vi "Date_to_Seconds.vi"() -> ()   [LabVIEW 2020]
panel:
  out "Resultat en second":dbl
  in  "Secondes":dbl
  in  "Minutes":dbl
  in  "Heures":dbl
  in  "Jours":dbl
  in  "Mois":dbl
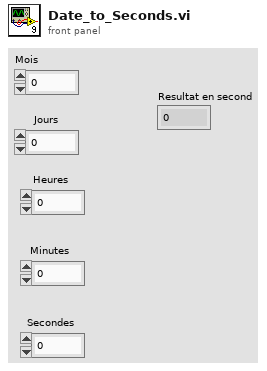
[diagram p1: front panel]
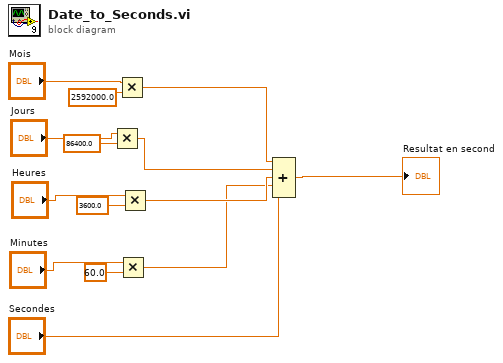
[diagram p0: block diagram]
diagram:
  n1 = Multiply(x="Jours", y=86400.0) -> (x*y=w5:dbl)
  n2 = Multiply(x="Mois", y=2592000.0) -> (x*y=w6:dbl)
  n3 = Multiply(x="Minutes", y=60.0) -> (x*y=w3:dbl)
  n4 = Multiply(x="Heures", y=3600.0) -> (x*y=w4:dbl)
  n5 = Compound Arithmetic op=ADD(w6, w5, w4, w3, "Secondes") -> (→"Resultat en second":dbl)
